vi "EllipsePerimeter.vi"(10 "a":dbl, 11 "b":dbl) -> (3 "Numeric":dbl)   [LabVIEW 2017, in "AODControl.lvlib"]
uses:
  AODControl.lvlib
  <vilib>/gmath/SpecialFunctions.llb/Complete Elliptic Integral E.vi
  <vilib>/gmath/NI_Gmath.lvlib
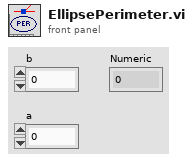
[diagram p1: front panel]
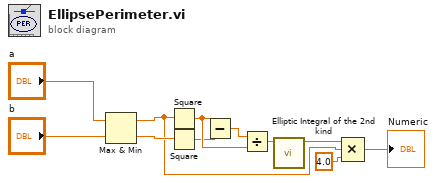
[diagram p0: block diagram]
diagram:
  n1 = Max & Min(x="a", y="b") -> (max(x,y)=w9:dbl, min(x,y)=w10:dbl)
  n2 = Square(x=w9) -> (x^2=w7:dbl)
  n3 = Square(x=w10) -> (x^2=w2:dbl)
  n4 = Subtract(x=w7, y=w2) -> (x-y=w3:dbl)
  n5 = Divide(x=w3, y=w7) -> (x/y=w8:dbl)
  n6 = call-poly <vilib>:"Elliptic Integral of the 2nd kind.vi"("k"=w8) -> ("E(k)"=w4:dbl)  [unwired: 10 in]
  n7 = Compound Arithmetic op=MULTIPLY(w4, w9, 4.0 ("value")) -> (→"Numeric":dbl)
